vi "stopHWError.vi"(8 "error in (no error)":errorcluster, 11 "AtomChipHWC in":refnum<class "AtomChipHWC.lvclass">) -> (0 "error out":errorcluster, 3 "AtomChipHWC out":refnum<class "AtomChipHWC.lvclass">)   [LabVIEW 2009, in "Hardware.lvlib" / "HWControllers.lvlib" / "AtomChipHWC.lvclass"]
uses:
  AtomChipHWC.lvclass
  HWController.lvclass
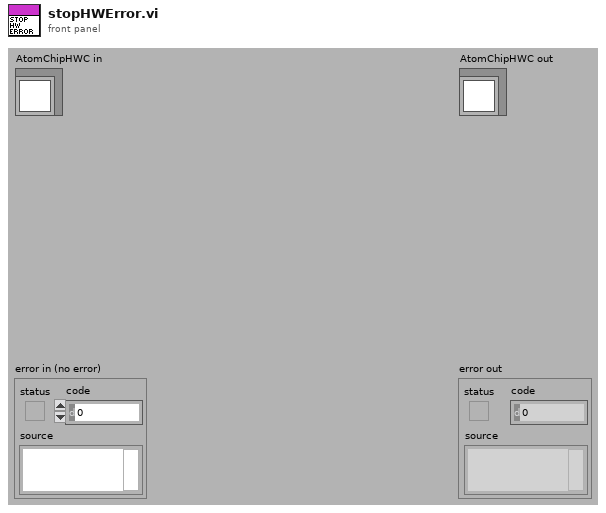
[diagram p1: front panel]
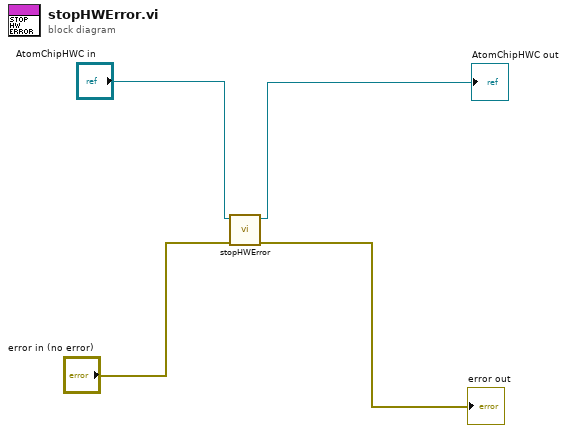
[diagram p0: block diagram]
diagram:
  n1 = call-parent "stopHWError.vi"("error in (no error)"="error in (no error)", "HWController in"="AtomChipHWC in") -> ("error out"=→"error out":errorcluster, "HWController out"=→"AtomChipHWC out":refnum<class "AtomChipHWC.lvclass">)  [unwired: 8 in]
